vi "DecimalNumToBinaryString.vi"(11 "十进制 整形":u32) -> (3 "二进制字符串":string)   [LabVIEW 2015]
doc: "本VI把十进制的数值转换为二进制的字符串输出"
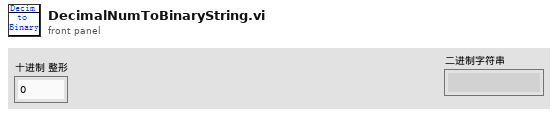
[diagram p1: front panel]
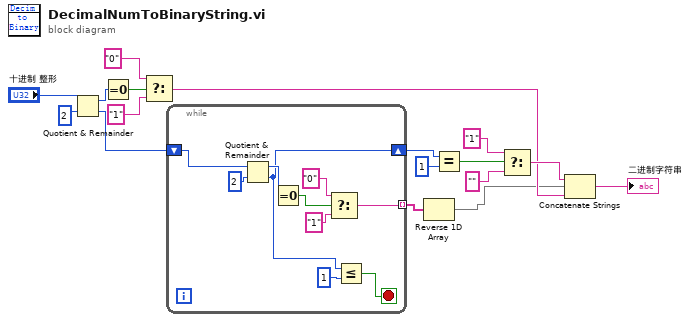
[diagram p0: block diagram]
diagram:
  n1 = Quotient & Remainder(x="十进制 整形", y=u32 2) -> (x-y*floor(x/y)=w9:u32, floor(x/y)=w15:u32)
  n2 = Equal To 0?(x=w9) -> (x = 0?=w6:bool)
  n3 = Select(t="0", s=w6, f="1") -> (s? t:f=w4:string)
  n4 = while {
    shift-right: [w20] -> w14
    shift-left: w15 -> [w27]
    tunnel: [w21] -> w3 mode=indexing
    stop <- w18 stop-if-true
    n5 = Quotient & Remainder(x=w27, y=u32 2) -> (x-y*floor(x/y)=w25:u32, floor(x/y)=w20:u32)
    n6 = Equal To 0?(x=w25) -> (x = 0?=w24:bool)
    n7 = Select(t="0", s=w24, f="1") -> (s? t:f=w21:string)
    n8 = Less Or Equal?(x=w20, y=u32 1) -> (x <= y?=w18:bool)
  }
  n9 = Reverse 1D Array(array=w3) -> (reversed array=w2:string[])
  n10 = Equal?(x=w14, y=u32 1) -> (x = y?=w12:bool)
  n11 = Select(t="1", s=w12, f="") -> (s? t:f=w5:string)
  n12 = Concatenate Strings(w5, w2, w4) -> (→"二进制字符串":string)
